vi "IDS Sort File Names.vi"(7 "Requested File Path":path) -> (8 "Resulting File Path":path)   [LabVIEW 2025]
uses:
  kernel32.dll
  shell32.dll
panel:
  out "ReName Success?":bool
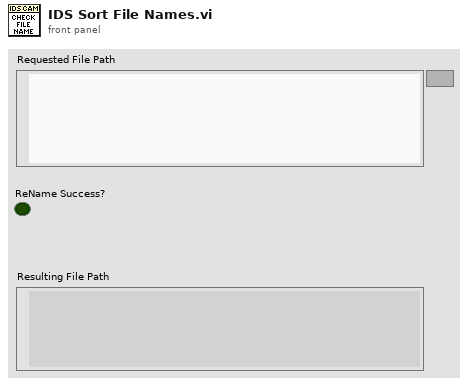
[diagram p1: front panel]
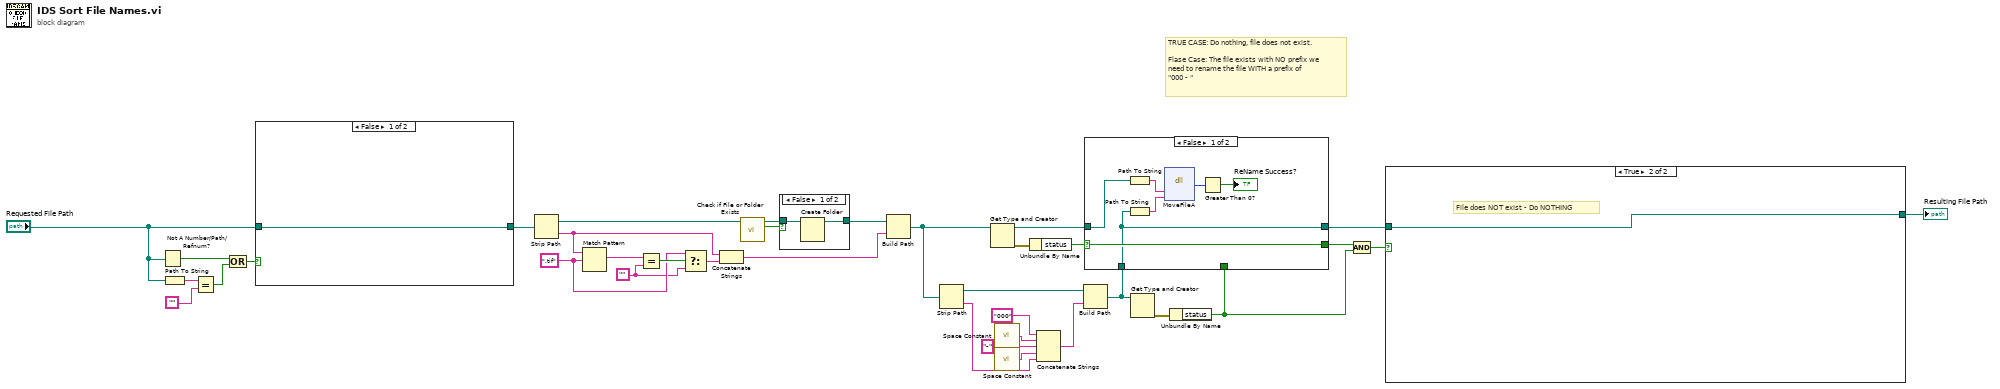
[diagram p0: block diagram]
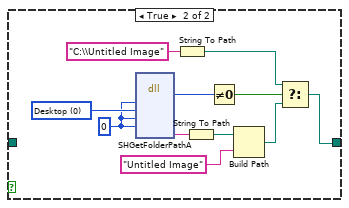
[diagram p3: hidden frame]
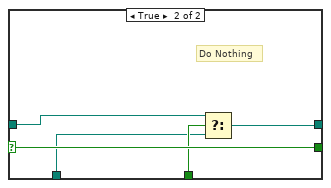
[diagram p4: hidden frame]
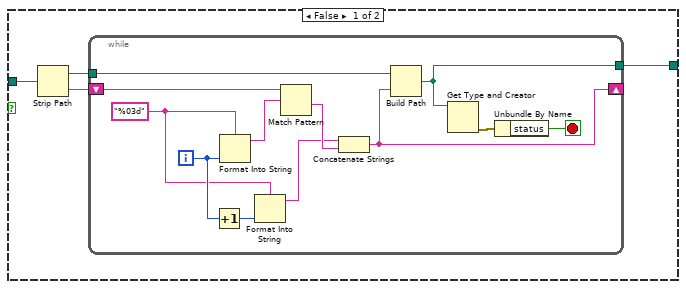
[diagram p5: hidden frame]
diagram:
  w14 = ""
  w15 = ".tif" ("regular expression")
  # "TRUE CASE: Do nothing, file does not exist.\n\nFlase Case: The file exists with NO prefix we\nneed to rename the file WITH a prefix of\n\"000 - \""
  n1 = Not A Number/Path/Refnum?(number/path/refnum="Requested File Path") -> (NaN/Path/Refnum?=w10:bool)
  n2 = Path To String(path="Requested File Path") -> (string=w12:string)
  n3 = Equal?(x=w12, y="") -> (x = y?=w9:bool)
  n4 = Or(x=w10, y=w9) -> (x .or. y?=w8:bool)
  n5 = case shown="False" w8 {
    tunnel: "Requested File Path" -> [w37 _]
    tunnel: [w37 w38] -> w6
    frame False {
    }
    frame True {
      w48 = 0 items=["Desktop"=0, "Personal Documents"=5, "AppData"=26, "Local AppData"=28, "Common AppData"=35, "Program Files"=38, "Program Files Common"=43, "Common Documents"=46] ("Requested Path")
      w47 = 0 ("HWND")
      n6 = dll-call lib="shell32.dll" fn="SHGetFolderPathA"("HWND"=w47, "nFolder"=w48, "hToken"=w47, "dwFlags"=w47) -> ("Succeeded"=w43:i32, "pszPath"=w46:string)  [unwired: 8 in, 2 out]
      n7 = String To Path(string="C:\\Untitled Image" ("regular expression")) -> (path=w40:path)
      n8 = String To Path(string=w46) -> (path=w45:path)
      n9 = Not Equal To 0?(x=w43) -> (x != 0?=w41:bool)
      n10 = Build Path(base path=w45, name or relative path="Untitled Image" ("regular expression")) -> (appended path=w39:path)
      n11 = Select(t=w40, s=w41, f=w39) -> (s? t:f=w38:path)
    }
  }
  n12 = Strip Path(path=w6) -> (stripped path=w2:path, name=w16:string)
  n13 = Match Pattern(string=w16, regular expression=w15) -> (match substring=w19:string)  [unwired: 1 in, 3 out]
  n14 = Equal?(x=w19, y=w14) -> (x = y?=w18:bool)
  n15 = Select(t=w15, s=w18, f=w14) -> (s? t:f=w17:string)
  n16 = Concatenate Strings(w16, w17) -> (w5:string)
  n17 = call <vilib>:"Check if File or Folder Exists.vi"("path"=w2) -> ("file or folder exists?"=w4:bool, "dup path"=w3:path)  [unwired: 8 in, 1 out]
  n18 = case shown="False" w4 {
    tunnel: [w49 w51] -> w1
    tunnel: w3 -> [w50 w51]
    frame False {
      n19 = Create Folder(path (use dialog)=w50) -> (created path=w49:path)  [unwired: 2 in, 2 out]
    }
    frame True {
    }
  }
  n20 = Build Path(base path=w1, name or relative path=w5) -> (appended path=w13:path)
  n21 = Strip Path(path=w13) -> (stripped path=w32:path, name=w28:string)
  n22 = Get Type and Creator(7:w13) -> (0:w35:errorcluster, 3:w23:path)  [unwired: 1 in, 2 out]
  n23 = call <vilib>:"Space Constant.vi"() -> ("String"=w34:string)
  n24 = call <vilib>:"Space Constant.vi"() -> ("String"=w30:string)
  n25 = Unbundle By Name(w35) -> ("status"=w25:bool)
  n26 = Concatenate Strings("000", w34, "-", w30, w28) -> (w31:string)
  n27 = Build Path(base path=w32, name or relative path=w31) -> (appended path=w21:path)
  n28 = Get Type and Creator(7:w21) -> (0:w27:errorcluster)  [unwired: 1 in, 3 out]
  n29 = Unbundle By Name(w27) -> ("status"=w20:bool)
  n30 = case shown="False" w25 {
    selector: w25 -> [w58 w63]
    tunnel: [w58 w63] -> w24
    tunnel: w23 -> [w53 w61]
    tunnel: [w52 w60] -> w22
    tunnel: w21 -> [w52 w59]
    tunnel: w20 -> [_ w62]
    frame False {
      n31 = Path To String(path=w53) -> (string=w55:string)
      n32 = Path To String(path=w52) -> (string=w54:string)
      n33 = dll-call lib="kernel32.dll" fn="MoveFileA"(w55, w54) -> ("return type"=w56:i32)  [unwired: 5 in, 2 out]
      n34 = Greater Than 0?(x=w56) -> (x > 0?=→"ReName Success?":bool)
    }
    frame True {
      # "Do Nothing"
      n35 = Select(t=w61, s=w62, f=w59) -> (s? t:f=w60:path)
    }
  }
  n36 = And(x=w24, y=w20) -> (x .and. y?=w26:bool)
  n37 = case shown="True" w26 {
    tunnel: w22 -> [w67 w80]
    tunnel: [w64 w80] -> w36
    frame False {
      n38 = Strip Path(path=w67) -> (stripped path=w66:path, name=w65:string)
      n39 = while {
        tunnel: w66 -> [w78]
        tunnel: [w75] -> w64
        shift-right: [w68] -> _
        shift-left: w65 -> [w79]
        i -> [w72]
        stop <- w73 stop-if-true
        w70 = "%03d" ("format string")
        n40 = Increment(x=w72) -> (x+1=w71:i32)
        n41 = Format Into String(format string=w70, w72) -> (resulting string=w77:string)  [unwired: 2 in, 1 out]
        n42 = Format Into String(format string=w70, w71) -> (resulting string=w69:string)  [unwired: 2 in, 1 out]
        n43 = Match Pattern(string=w79, regular expression=w77) -> (after substring=w76:string)  [unwired: 1 in, 3 out]
        n44 = Concatenate Strings(w69, w76) -> (w68:string)
        n45 = Build Path(base path=w78, name or relative path=w68) -> (appended path=w75:path)
        n46 = Get Type and Creator(7:w75) -> (0:w74:errorcluster)  [unwired: 1 in, 3 out]
        n47 = Unbundle By Name(w74) -> ("status"=w73:bool)
      }
    }
    frame True {
      # "File does NOT exist - Do NOTHING"
    }
  }
  "Resulting File Path" <- w36
